vi "Message Packet To String.vi"(8 "error in (no error)":errorcluster, 11 "Message Packet":variant) -> (0 "error out":errorcluster, 3 "String":string)   [LabVIEW 2020, in "SECS Communication.lvlib" / "HSMS Class.lvclass"]
uses:
  HSMS Class.lvclass
  Message Packet.ctl
  Message Header.ctl
  PType.ctl
  SType.ctl
  SECS-II Class/SECS-II Class.lvclass
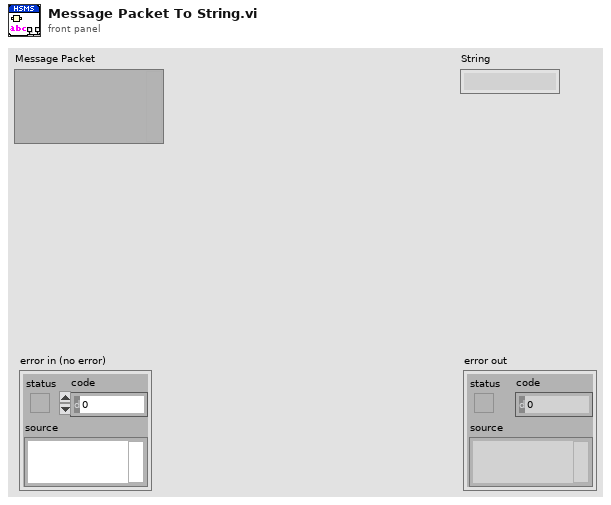
[diagram p1: front panel]
types:
  T1 = typedef "SECS Communication.lvlib/HSMS Class.lvclass/Message Packet.ctl" = cluster{"Message Header Cluster":T2, "Message Header":u8[], "Message Text":u8[]}
  T2 = typedef "SECS Communication.lvlib/HSMS Class.lvclass/Message Header.ctl" = cluster{"Byte 0-1(Session ID)":u16, "W-Bit":bool, "Byte 2":u8, "Byte 3":u8, "Byte 4(PType)":T3, "Byte 5(SType)":T4, "Byte 6-9(System Btyes)":u8[]}
  T3 = typedef "SECS Communication.lvlib/HSMS Class.lvclass/PType.ctl" = enum8{"SECS-II Encoding", "Reserved"}
  T4 = typedef "SECS Communication.lvlib/HSMS Class.lvclass/SType.ctl" = enum8{"Data Message", "Select.req", "Select.rsp", "Deselect.req", "Deselect.rsp", "Linktest.req", "Linktest.rsp", "Reject.req", "Separate.req"}
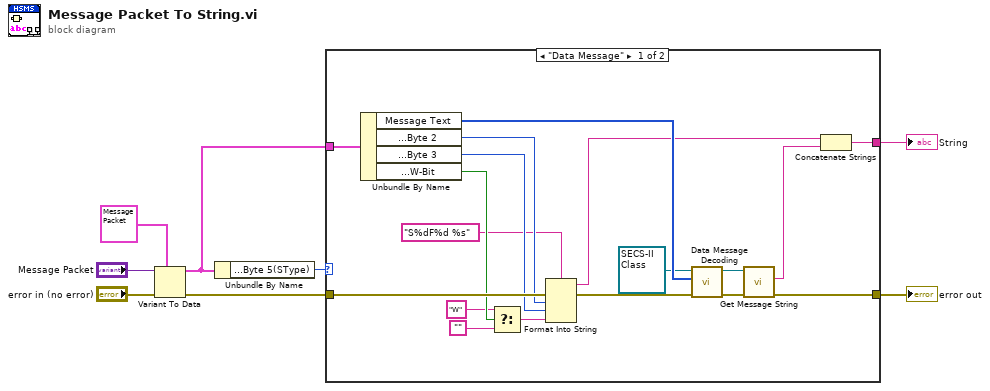
[diagram p0: block diagram]
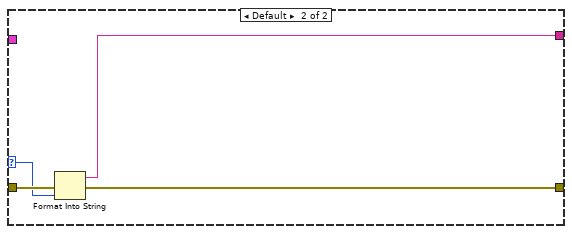
[diagram p2: hidden frame]
diagram:
  n1 = Variant To Data(error in="error in (no error)", type=T1 {"Message Header Cluster"={"Byte 0-1(Session ID)"=0, "W-Bit"=FALSE, "Byte 2"=0, "Byte 3"=0, "Byte 4(PType)"=enum."SECS-II Encoding", "Byte 5(SType)"=enum."Data Message", "Byte 6-9(System Btyes)"=[]}, "Message Header"=[], "Message Text"=[]} ("Message Packet"), Variant="Message Packet") -> (data=w3:T1, error out=w5:errorcluster)
  n2 = Unbundle By Name(w3) -> ("Message Header Cluster.Byte 5(SType)"=w4:T4)
  n3 = case shown="\"Data Message\"" w4 {
    selector: w4 -> [_ w29]
    tunnel: w5 -> [w25 w30]
    tunnel: w3 -> [w26 _]
    tunnel: [w9 w28] -> w2
    tunnel: [w10 w27] -> w1
    frame "Data Message" {
      n4 = Unbundle By Name(w26) -> ("Message Text"=w17:u8[], "Message Header Cluster.Byte 2"=w23:u8, "Message Header Cluster.Byte 3"=w24:u8, "Message Header Cluster.W-Bit"=w22:bool)
      n5 = Select(t="W", s=w22, f="") -> (s? t:f=w19:string)
      n6 = Format Into String(format string="S%dF%d %s", error in=w25, w23, w24, w19) -> (resulting string=w12:string, error out=w18:errorcluster)  [unwired: 1 in]
      n7 = call "Data Message Decoding.vi"("error in"=w18, "Message Text"=w17, "SECS-II Class in"=refnum<class "SECS-II Class.lvclass"> refnum) -> ("error out"=w14:errorcluster, "SECS-II Class out"=w13:refnum<class "SECS-II Class.lvclass">)  [unwired: 6 in, 1 out]
      n8 = call "Get Message String.vi"("error in (no error)"=w14, "SECS-II Class in"=w13) -> ("error out"=w9:errorcluster, "String"=w11:string)  [unwired: 7 in, 1 out]
      n9 = Concatenate Strings(w12, w11) -> (w10:string)
    }
    frame Default {
      n10 = Format Into String(error in=w30, w29) -> (resulting string=w27:string, error out=w28:errorcluster)  [unwired: 2 in]
    }
  }
  "error out" <- w2
  "String" <- w1
